vi "FTW-STR-Encode-Base64.vi"(0 "Input":string, 1 "Direction":enum16{"Encode", "Decode"}(ring)) -> (2 "Output":string)   [LabVIEW 2013]
panel:
  # "Inputs"
  # "Outputs"
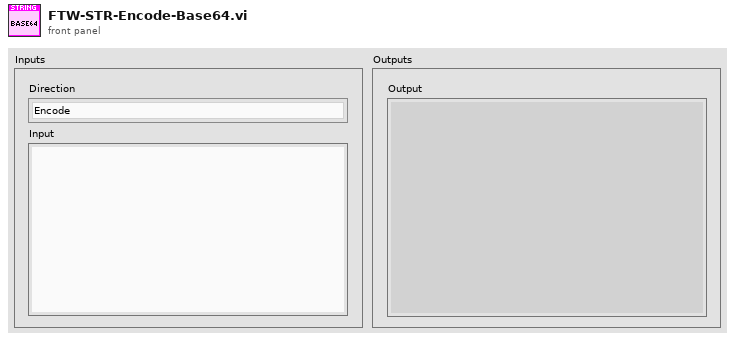
[diagram p1: front panel]
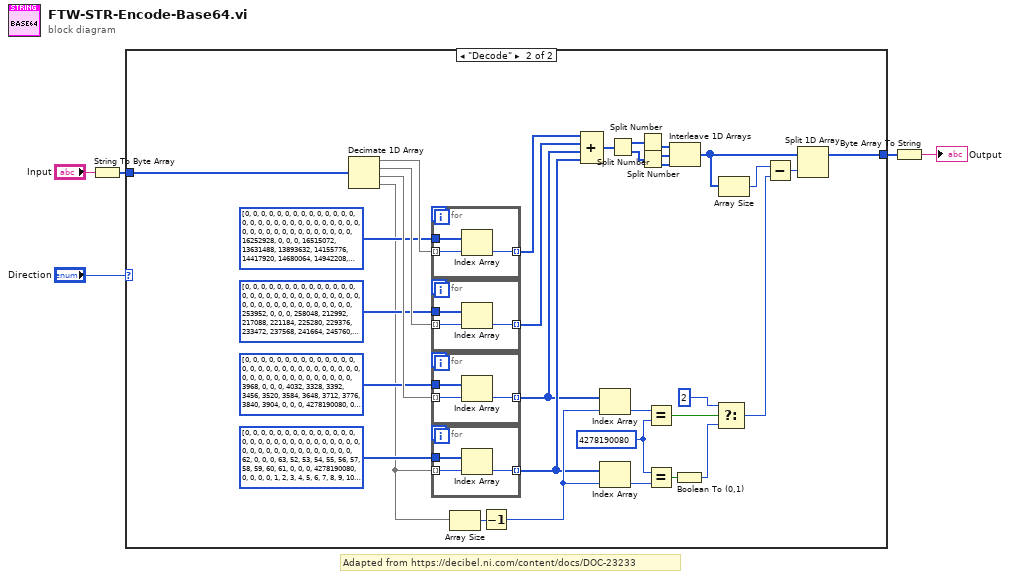
[diagram p0: block diagram]
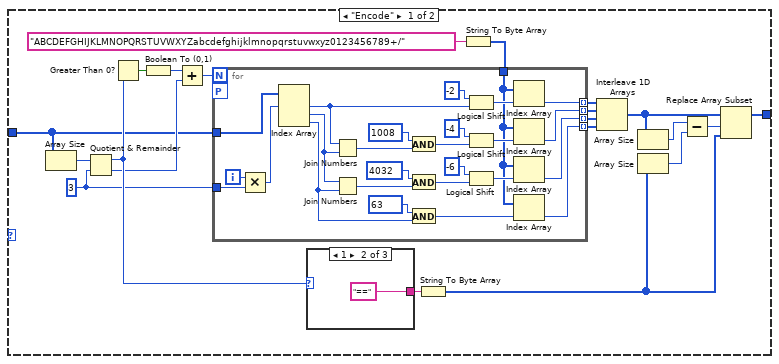
[diagram p2: hidden frame]
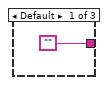
[diagram p3: hidden frame]
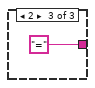
[diagram p4: hidden frame]
diagram:
  # "Adapted from https://decibel.ni.com/content/docs/DOC-23233"
  n1 = String To Byte Array(string="Input") -> (unsigned byte array=w1:u8[])
  n2 = case shown="\"Decode\"" "Direction" {
    tunnel: [w7 w57] -> w4
    tunnel: w1 -> [w6 w56]
    frame "Encode" {
      w12 = 3 ("y")
      n3 = Array Size(array=w6) -> (size(s)=w22:i32)
      n4 = Quotient & Remainder(x=w22, y=w12) -> (x-y*floor(x/y)=w18:i32, floor(x/y)=w11:i32)
      n5 = Greater Than 0?(x=w18) -> (x > 0?=w9:bool)
      n6 = Boolean To (0,1)(Boolean=w9) -> (0, 1=w8:i16)
      n7 = Add(x=w8, y=w11) -> (x+y=w10:i32)
      n8 = case shown="1" w18 {
        tunnel: ["" "==" "="] -> w17
        frame Default {
        }
        frame 1 {
        }
        frame 2 {
        }
      }
      n9 = String To Byte Array(string=w17) -> (unsigned byte array=w13:u8[])
      n10 = String To Byte Array(string="ABCDEFGHIJKLMNOPQRSTUVWXYZabcdefghijklmnopqrstuvwxyz0123456789+/") -> (unsigned byte array=w20:u8[])
      n11 = for {
        N: w10 -> [_]
        tunnel: [w38] -> w26 mode=indexing
        tunnel: [w39] -> w25 mode=indexing
        tunnel: [w40] -> w24 mode=indexing
        tunnel: [w41] -> w23 mode=indexing
        workers-P: _ -> [_]
        tunnel: w20 -> [w34]
        tunnel: w12 -> [w32]
        tunnel: w6 -> [w30]
        i -> [w33]
        n12 = Multiply(x=w33, y=w32) -> (x*y=w31:i32)
        n13 = Index Array(array=w30, index #1=w31) -> (element #1=w37:u8, element #2=w36:u8, element #3=w35:u8)  [unwired: 2 in]
        n14 = Join Numbers(hi=w37, lo=w36) -> ((hi.lo)=w54:u16)
        n15 = Join Numbers(hi=w36, lo=w35) -> ((hi.lo)=w50:u16)
        n16 = And(x=u16 1008, y=w54) -> (x .and. y?=w52:u16)
        n17 = And(x=u16 4032, y=w50) -> (x .and. y?=w48:u16)
        n18 = And(x=u8 63, y=w35) -> (x .and. y?=w42:u8)
        n19 = Logical Shift(y=i8 -2, x=w37) -> (x << y=w45:u8)
        n20 = Logical Shift(y=i8 -4, x=w52) -> (x << y=w44:u16)
        n21 = Logical Shift(y=i8 -6, x=w48) -> (x << y=w43:u16)
        n22 = Index Array(array=w34, index=w45) -> (element=w41:u8)
        n23 = Index Array(array=w34, index=w44) -> (element=w40:u8)
        n24 = Index Array(array=w34, index=w43) -> (element=w39:u8)
        n25 = Index Array(array=w34, index=w42) -> (element=w38:u8)
      }
      n26 = Interleave 1D Arrays(w23, w24, w25, w26) -> (w19:u8[])
      n27 = Array Size(array=w19) -> (size(s)=w15:i32)
      n28 = Array Size(array=w13) -> (size(s)=w14:i32)
      n29 = Subtract(x=w15, y=w14) -> (x-y=w16:i32)
      n30 = Replace Array Subset(array=w19, new element=w13, index=w16) -> (w7:u8[])
    }
    frame "Decode" {
      w78 = u32 4278190080 ("y")
      n31 = Decimate 1D Array(w56) -> (w73:u8[], w75:u8[], w77:u8[], w66:u8[])
      n32 = for {
        tunnel: u32[] [0, 0, 0, 0, 0, 0, 0, 0, 0, 0, 0, 0, 0, 0, 0, 0, 0, 0, 0, 0, 0, 0, 0, 0, 0, 0, 0, 0, 0, 0, 0, 0, 0, 0, 0, 0, 0, 0, 0, 0, 0, 0, 0, 16252928, 0, 0, 0, 16515072, 13631488, 13893632, 14155776, 14417920, 14680064, 14942208, 15204352, 15466496, 15728640, 15990784, 0, 0, 0, 0, 0, 0, 0, 0, 262144, 524288, 786432, 1048576, 1310720, 1572864, 1835008, 2097152, 2359296, 2621440, 2883584, 3145728, 3407872, 3670016, 3932160, 4194304, 4456448, 4718592, 4980736, 5242880, 5505024, 5767168, 6029312, 6291456, 6553600, 0, 0, 0, 0, 0, 0, 6815744, 7077888, 7340032, 7602176, 7864320, 8126464, 8388608, 8650752, 8912896, 9175040, 9437184, 9699328, 9961472, 10223616, 10485760, 10747904, 11010048, 11272192, 11534336, 11796480, 12058624, 12320768, 12582912, 12845056, 13107200, 13369344, 0, 0, 0, 0, 0, 0, 0, 0, 0, 0, 0, 0, 0, 0, 0, 0, 0, 0, 0, 0, 0, 0, 0, 0, 0, 0, 0, 0, 0, 0, 0, 0, 0, 0, 0, 0, 0, 0, 0, 0, 0, 0, 0, 0, 0, 0, 0, 0, 0, 0, 0, 0, 0, 0, 0, 0, 0, 0, 0, 0, 0, 0, 0, 0, 0, 0, 0, 0, 0, 0, 0, 0, 0, 0, 0, 0, 0, 0, 0, 0, 0, 0, 0, 0, 0, 0, 0, 0, 0, 0, 0, 0, 0, 0, 0, 0, 0, 0, 0, 0, 0, 0, 0, 0, 0, 0, 0, 0, 0, 0, 0, 0, 0, 0, 0, 0, 0, 0, 0, 0, 0, 0, 0, 0, 0, 0, 0, 0, 0, 0, 0, 0, 0] ("array 4") -> [w91]
        tunnel: [w90] -> w72 mode=indexing
        tunnel: w73 -> [w89] mode=indexing
        n33 = Index Array(array=w91, index=w89) -> (element=w90:u32)
      }
      n34 = for {
        tunnel: u32[] [0, 0, 0, 0, 0, 0, 0, 0, 0, 0, 0, 0, 0, 0, 0, 0, 0, 0, 0, 0, 0, 0, 0, 0, 0, 0, 0, 0, 0, 0, 0, 0, 0, 0, 0, 0, 0, 0, 0, 0, 0, 0, 0, 253952, 0, 0, 0, 258048, 212992, 217088, 221184, 225280, 229376, 233472, 237568, 241664, 245760, 249856, 0, 0, 0, 0, 0, 0, 0, 0, 4096, 8192, 12288, 16384, 20480, 24576, 28672, 32768, 36864, 40960, 45056, 49152, 53248, 57344, 61440, 65536, 69632, 73728, 77824, 81920, 86016, 90112, 94208, 98304, 102400, 0, 0, 0, 0, 0, 0, 106496, 110592, 114688, 118784, 122880, 126976, 131072, 135168, 139264, 143360, 147456, 151552, 155648, 159744, 163840, 167936, 172032, 176128, 180224, 184320, 188416, 192512, 196608, 200704, 204800, 208896, 0, 0, 0, 0, 0, 0, 0, 0, 0, 0, 0, 0, 0, 0, 0, 0, 0, 0, 0, 0, 0, 0, 0, 0, 0, 0, 0, 0, 0, 0, 0, 0, 0, 0, 0, 0, 0, 0, 0, 0, 0, 0, 0, 0, 0, 0, 0, 0, 0, 0, 0, 0, 0, 0, 0, 0, 0, 0, 0, 0, 0, 0, 0, 0, 0, 0, 0, 0, 0, 0, 0, 0, 0, 0, 0, 0, 0, 0, 0, 0, 0, 0, 0, 0, 0, 0, 0, 0, 0, 0, 0, 0, 0, 0, 0, 0, 0, 0, 0, 0, 0, 0, 0, 0, 0, 0, 0, 0, 0, 0, 0, 0, 0, 0, 0, 0, 0, 0, 0, 0, 0, 0, 0, 0, 0, 0, 0, 0, 0, 0, 0, 0, 0] ("array 3") -> [w94]
        tunnel: [w93] -> w74 mode=indexing
        tunnel: w75 -> [w92] mode=indexing
        n35 = Index Array(array=w94, index=w92) -> (element=w93:u32)
      }
      n36 = for {
        tunnel: u32[] [0, 0, 0, 0, 0, 0, 0, 0, 0, 0, 0, 0, 0, 0, 0, 0, 0, 0, 0, 0, 0, 0, 0, 0, 0, 0, 0, 0, 0, 0, 0, 0, 0, 0, 0, 0, 0, 0, 0, 0, 0, 0, 0, 3968, 0, 0, 0, 4032, 3328, 3392, 3456, 3520, 3584, 3648, 3712, 3776, 3840, 3904, 0, 0, 0, 4278190080, 0, 0, 0, 0, 64, 128, 192, 256, 320, 384, 448, 512, 576, 640, 704, 768, 832, 896, 960, 1024, 1088, 1152, 1216, 1280, 1344, 1408, 1472, 1536, 1600, 0, 0, 0, 0, 0, 0, 1664, 1728, 1792, 1856, 1920, 1984, 2048, 2112, 2176, 2240, 2304, 2368, 2432, 2496, 2560, 2624, 2688, 2752, 2816, 2880, 2944, 3008, 3072, 3136, 3200, 3264, 0, 0, 0, 0, 0, 0, 0, 0, 0, 0, 0, 0, 0, 0, 0, 0, 0, 0, 0, 0, 0, 0, 0, 0, 0, 0, 0, 0, 0, 0, 0, 0, 0, 0, 0, 0, 0, 0, 0, 0, 0, 0, 0, 0, 0, 0, 0, 0, 0, 0, 0, 0, 0, 0, 0, 0, 0, 0, 0, 0, 0, 0, 0, 0, 0, 0, 0, 0, 0, 0, 0, 0, 0, 0, 0, 0, 0, 0, 0, 0, 0, 0, 0, 0, 0, 0, 0, 0, 0, 0, 0, 0, 0, 0, 0, 0, 0, 0, 0, 0, 0, 0, 0, 0, 0, 0, 0, 0, 0, 0, 0, 0, 0, 0, 0, 0, 0, 0, 0, 0, 0, 0, 0, 0, 0, 0, 0, 0, 0, 0, 0, 0, 0] ("array 2") -> [w97]
        tunnel: [w96] -> w76 mode=indexing
        tunnel: w77 -> [w95] mode=indexing
        n37 = Index Array(array=w97, index=w95) -> (element=w96:u32)
      }
      n38 = for {
        tunnel: u32[] [0, 0, 0, 0, 0, 0, 0, 0, 0, 0, 0, 0, 0, 0, 0, 0, 0, 0, 0, 0, 0, 0, 0, 0, 0, 0, 0, 0, 0, 0, 0, 0, 0, 0, 0, 0, 0, 0, 0, 0, 0, 0, 0, 62, 0, 0, 0, 63, 52, 53, 54, 55, 56, 57, 58, 59, 60, 61, 0, 0, 0, 4278190080, 0, 0, 0, 0, 1, 2, 3, 4, 5, 6, 7, 8, 9, 10, 11, 12, 13, 14, 15, 16, 17, 18, 19, 20, 21, 22, 23, 24, 25, 0, 0, 0, 0, 0, 0, 26, 27, 28, 29, 30, 31, 32, 33, 34, 35, 36, 37, 38, 39, 40, 41, 42, 43, 44, 45, 46, 47, 48, 49, 50, 51, 0, 0, 0, 0, 0, 0, 0, 0, 0, 0, 0, 0, 0, 0, 0, 0, 0, 0, 0, 0, 0, 0, 0, 0, 0, 0, 0, 0, 0, 0, 0, 0, 0, 0, 0, 0, 0, 0, 0, 0, 0, 0, 0, 0, 0, 0, 0, 0, 0, 0, 0, 0, 0, 0, 0, 0, 0, 0, 0, 0, 0, 0, 0, 0, 0, 0, 0, 0, 0, 0, 0, 0, 0, 0, 0, 0, 0, 0, 0, 0, 0, 0, 0, 0, 0, 0, 0, 0, 0, 0, 0, 0, 0, 0, 0, 0, 0, 0, 0, 0, 0, 0, 0, 0, 0, 0, 0, 0, 0, 0, 0, 0, 0, 0, 0, 0, 0, 0, 0, 0, 0, 0, 0, 0, 0, 0, 0, 0, 0, 0, 0, 0, 0] ("Array") -> [w100]
        tunnel: [w99] -> w80 mode=indexing
        tunnel: w66 -> [w98] mode=indexing
        n39 = Index Array(array=w100, index=w98) -> (element=w99:u32)
      }
      n40 = Array Size(array=w66) -> (size(s)=w82:i32)
      n41 = Decrement(x=w82) -> (x-1=w81:i32)
      n42 = Compound Arithmetic op=ADD(w72, w74, w76, w80) -> (w87:u32[])
      n43 = Index Array(array=w76, index=w81) -> (element=w79:u32)
      n44 = Index Array(array=w80, index=w81) -> (element=w60:u32)
      n45 = Split Number(x=w87) -> (hi(x)=w88:u16[], lo(x)=w86:u16[])
      n46 = Split Number(x=w88) -> (lo(x)=w83:u8[])  [unwired: 1 out]
      n47 = Split Number(x=w86) -> (hi(x)=w84:u8[], lo(x)=w85:u8[])
      n48 = Equal?(x=w79, y=w78) -> (x = y?=w63:bool)
      n49 = Equal?(x=w78, y=w60) -> (x = y?=w59:bool)
      n50 = Interleave 1D Arrays(w83, w84, w85) -> (w67:u8[])
      n51 = Boolean To (0,1)(Boolean=w59) -> (0, 1=w61:i16)
      n52 = Select(t=2, s=w63, f=w61) -> (s? t:f=w58:i32)
      n53 = Array Size(array=w67) -> (size(s)=w64:i32)
      n54 = Subtract(x=w64, y=w58) -> (x-y=w65:i32)
      n55 = Split 1D Array(array=w67, index=w65) -> (first subarray=w57:u8[])  [unwired: 1 out]
    }
  }
  n56 = Byte Array To String(unsigned byte array=w4) -> (string=→"Output":string)
